vi "Host Child.vi"(0 "LV MDI in":refnum<class "LV MDI.lvclass">, 5 "Child Hwnd":u32, 11 "error in (no error)":errorcluster) -> (4 "LV MDI out":refnum<class "LV MDI.lvclass">, 15 "error out":errorcluster)   [LabVIEW 2016, in "LV MDI.lvclass"]
doc: "Changes parent window of specified child."
uses:
  LV MDI.lvclass
  LV MDI.lvclass/LV MDI.ctl
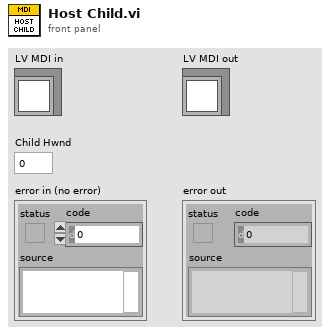
[diagram p1: front panel]
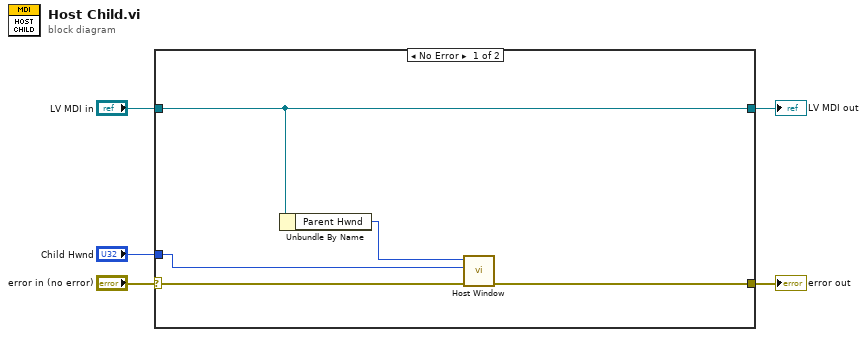
[diagram p0: block diagram]
diagram:
  n1 = case shown="No Error" "error in (no error)" {
    selector: "error in (no error)" -> [w10 w12]
    tunnel: [w6 w12] -> w4
    tunnel: [w8 w11] -> w2
    tunnel: "LV MDI in" -> [w8 w11]
    tunnel: "Child Hwnd" -> [w7 _]
    frame No Error {
      n2 = Unbundle By Name(w8) -> ("Parent Hwnd"=w9:i32)
      n3 = call "Host Window.vi"("error in (no error)"=w10, "Child Hwnd"=w7, "Parent Hwnd"=w9) -> ("error out"=w6:errorcluster)  [unwired: 8 in]
    }
    frame Error {
    }
  }
  "error out" <- w4
  "LV MDI out" <- w2
